vi "Get Disable.vi"(8 "error in (no error)":errorcluster, 11 "S4ACS_GUI in":refnum<class "S4ACS_GUI.lvclass">) -> (0 "error out":errorcluster, 2 "Cluster Disable":T1, 3 "S4ACS_GUI out":refnum<class "S4ACS_GUI.lvclass">)   [LabVIEW 2018, in "S4ACS_GUI.lvclass"]
uses:
  S4ACS_GUI.lvclass
  S4ACS_GUI.lvclass/S4ACS_GUI.ctl
  Acquisition/Acquisition.lvclass
  Instrument/Instrument.lvclass
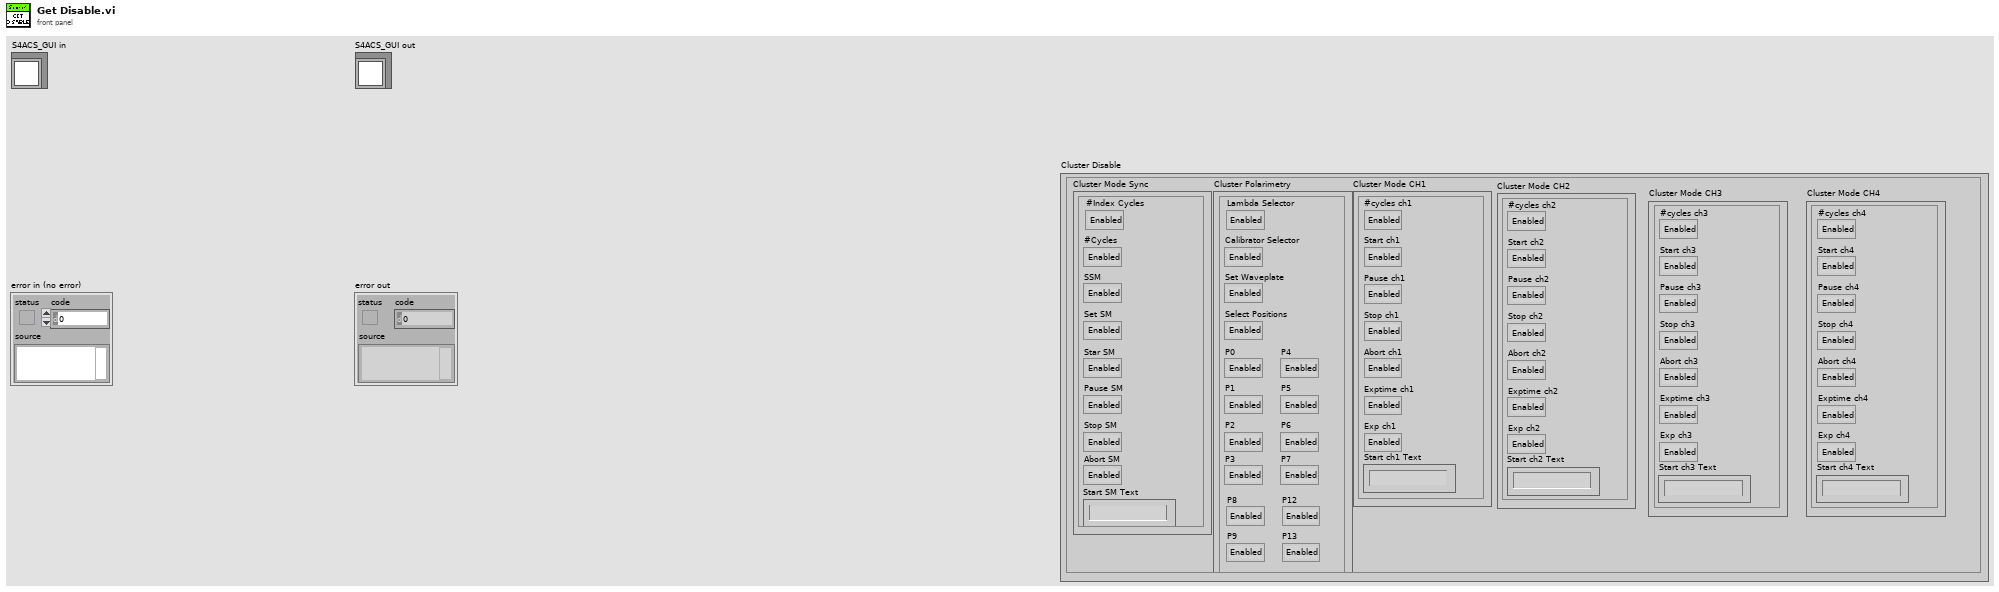
[diagram p1: front panel]
types:
  T1 = cluster{"Cluster Mode Sync":cluster{"#Index Cycles":enum8{"Enabled", "Disabled", "Disabled and Grayed Out"}, "#Cycles":enum8{"Enabled", "Disabled", "Disabled and Grayed Out"}, "SSM":enum8{"Enabled", "Disabled", "Disabled and Grayed Out"}, "Set SM":enum8{"Enabled", "Disabled", "Disabled and Grayed Out"}, "Star SM":enum8{"Enabled", "Disabled", "Disabled and Grayed Out"}, "Pause SM":enum8{"Enabled", "Disabled", "Disabled and Grayed Out"}, "Stop SM":enum8{"Enabled", "Disabled", "Disabled and Grayed Out"}, "Abort SM":enum8{"Enabled", "Disabled", "Disabled and Grayed Out"}, "Start SM Text":string}, "Cluster Polarimetry":cluster{"Lambda Selector":enum8{"Enabled", "Disabled", "Disabled and Grayed Out"}, "Calibrator Selector":enum8{"Enabled", "Disabled", "Disabled and Grayed Out"}, "Set Waveplate":enum8{"Enabled", "Disabled", "Disabled and Grayed Out"}, "Select Positions":enum8{"Enabled", "Disabled", "Disabled and Grayed Out"}, "P0":enum8{"Enabled", "Disabled", "Disabled and Grayed Out"}, "P1":enum8{"Enabled", "Disabled", "Disabled and Grayed Out"}, "P2":enum8{"Enabled", "Disabled", "Disabled and Grayed Out"}, "P3":enum8{"Enabled", "Disabled", "Disabled and Grayed Out"}, "P4":enum8{"Enabled", "Disabled", "Disabled and Grayed Out"}, "P5":enum8{"Enabled", "Disabled", "Disabled and Grayed Out"}, "P6":enum8{"Enabled", "Disabled", "Disabled and Grayed Out"}, "P7":enum8{"Enabled", "Disabled", "Disabled and Grayed Out"}, "P8":enum8{"Enabled", "Disabled", "Disabled and Grayed Out"}, "P9":enum8{"Enabled", "Disabled", "Disabled and Grayed Out"}, "P10":enum8{"Enabled", "Disabled", "Disabled and Grayed Out"}, "P11":enum8{"Enabled", "Disabled", "Disabled and Grayed Out"}, "P12":enum8{"Enabled", "Disabled", "Disabled and Grayed Out"}, "P13":enum8{"Enabled", "Disabled", "Disabled and Grayed Out"}, "P14":enum8{"Enabled", "Disabled", "Disabled and Grayed Out"}, "P15":enum8{"Enabled", "Disabled", "Disabled and Grayed Out"}}, "Cluster Mode CH1":cluster{"#cycles ch1":enum8{"Enabled", "Disabled", "Disabled and Grayed Out"}, "Start ch1":enum8{"Enabled", "Disabled", "Disabled and Grayed Out"}, "Pause ch1":enum8{"Enabled", "Disabled", "Disabled and Grayed Out"}, "Stop ch1":enum8{"Enabled", "Disabled", "Disabled and Grayed Out"}, "Abort ch1":enum8{"Enabled", "Disabled", "Disabled and Grayed Out"}, "Exptime ch1":enum8{"Enabled", "Disabled", "Disabled and Grayed Out"}, "Exp ch1":enum8{"Enabled", "Disabled", "Disabled and Grayed Out"}, "Start ch1 Text":string}, "Cluster Mode CH2":cluster{"#cycles ch2":enum8{"Enabled", "Disabled", "Disabled and Grayed Out"}, "Start ch2":enum8{"Enabled", "Disabled", "Disabled and Grayed Out"}, "Pause ch2":enum8{"Enabled", "Disabled", "Disabled and Grayed Out"}, "Stop ch2":enum8{"Enabled", "Disabled", "Disabled and Grayed Out"}, "Abort ch2":enum8{"Enabled", "Disabled", "Disabled and Grayed Out"}, "Exptime ch2":enum8{"Enabled", "Disabled", "Disabled and Grayed Out"}, "Exp ch2":enum8{"Enabled", "Disabled", "Disabled and Grayed Out"}, "Start ch2 Text":string}, "Cluster Mode CH3":cluster{"#cycles ch3":enum8{"Enabled", "Disabled", "Disabled and Grayed Out"}, "Start ch3":enum8{"Enabled", "Disabled", "Disabled and Grayed Out"}, "Pause ch3":enum8{"Enabled", "Disabled", "Disabled and Grayed Out"}, "Stop ch3":enum8{"Enabled", "Disabled", "Disabled and Grayed Out"}, "Abort ch3":enum8{"Enabled", "Disabled", "Disabled and Grayed Out"}, "Exptime ch3":enum8{"Enabled", "Disabled", "Disabled and Grayed Out"}, "Exp ch3":enum8{"Enabled", "Disabled", "Disabled and Grayed Out"}, "Start ch3 Text":string}, "Cluster Mode CH4":cluster{"#cycles ch4":enum8{"Enabled", "Disabled", "Disabled and Grayed Out"}, "Start ch4":enum8{"Enabled", "Disabled", "Disabled and Grayed Out"}, "Pause ch4":enum8{"Enabled", "Disabled", "Disabled and Grayed Out"}, "Stop ch4":enum8{"Enabled", "Disabled", "Disabled and Grayed Out"}, "Abort ch4":enum8{"Enabled", "Disabled", "Disabled and Grayed Out"}, "Exptime ch4":enum8{"Enabled", "Disabled", "Disabled and Grayed Out"}, "Exp ch4":enum8{"Enabled", "Disabled", "Disabled and Grayed Out"}, "Start ch4 Text":string}}
  T2 = enum8{"Enabled", "Disabled", "Disabled and Grayed Out"}
  T3 = cluster{"#Index Cycles":enum8{"Enabled", "Disabled", "Disabled and Grayed Out"}, "#Cycles":enum8{"Enabled", "Disabled", "Disabled and Grayed Out"}, "SSM":enum8{"Enabled", "Disabled", "Disabled and Grayed Out"}, "Set SM":enum8{"Enabled", "Disabled", "Disabled and Grayed Out"}, "Star SM":enum8{"Enabled", "Disabled", "Disabled and Grayed Out"}, "Pause SM":enum8{"Enabled", "Disabled", "Disabled and Grayed Out"}, "Stop SM":enum8{"Enabled", "Disabled", "Disabled and Grayed Out"}, "Abort SM":enum8{"Enabled", "Disabled", "Disabled and Grayed Out"}, "Start SM Text":string}
  T4 = cluster{"#cycles ch1":enum8{"Enabled", "Disabled", "Disabled and Grayed Out"}, "Start ch1":enum8{"Enabled", "Disabled", "Disabled and Grayed Out"}, "Pause ch1":enum8{"Enabled", "Disabled", "Disabled and Grayed Out"}, "Stop ch1":enum8{"Enabled", "Disabled", "Disabled and Grayed Out"}, "Abort ch1":enum8{"Enabled", "Disabled", "Disabled and Grayed Out"}, "Exptime ch1":enum8{"Enabled", "Disabled", "Disabled and Grayed Out"}, "Exp ch1":enum8{"Enabled", "Disabled", "Disabled and Grayed Out"}, "Start ch1 Text":string}
  T5 = cluster{"#cycles ch2":enum8{"Enabled", "Disabled", "Disabled and Grayed Out"}, "Start ch2":enum8{"Enabled", "Disabled", "Disabled and Grayed Out"}, "Pause ch2":enum8{"Enabled", "Disabled", "Disabled and Grayed Out"}, "Stop ch2":enum8{"Enabled", "Disabled", "Disabled and Grayed Out"}, "Abort ch2":enum8{"Enabled", "Disabled", "Disabled and Grayed Out"}, "Exptime ch2":enum8{"Enabled", "Disabled", "Disabled and Grayed Out"}, "Exp ch2":enum8{"Enabled", "Disabled", "Disabled and Grayed Out"}, "Start ch2 Text":string}
  T6 = cluster{"#cycles ch3":enum8{"Enabled", "Disabled", "Disabled and Grayed Out"}, "Start ch3":enum8{"Enabled", "Disabled", "Disabled and Grayed Out"}, "Pause ch3":enum8{"Enabled", "Disabled", "Disabled and Grayed Out"}, "Stop ch3":enum8{"Enabled", "Disabled", "Disabled and Grayed Out"}, "Abort ch3":enum8{"Enabled", "Disabled", "Disabled and Grayed Out"}, "Exptime ch3":enum8{"Enabled", "Disabled", "Disabled and Grayed Out"}, "Exp ch3":enum8{"Enabled", "Disabled", "Disabled and Grayed Out"}, "Start ch3 Text":string}
  T7 = cluster{"#cycles ch4":enum8{"Enabled", "Disabled", "Disabled and Grayed Out"}, "Start ch4":enum8{"Enabled", "Disabled", "Disabled and Grayed Out"}, "Pause ch4":enum8{"Enabled", "Disabled", "Disabled and Grayed Out"}, "Stop ch4":enum8{"Enabled", "Disabled", "Disabled and Grayed Out"}, "Abort ch4":enum8{"Enabled", "Disabled", "Disabled and Grayed Out"}, "Exptime ch4":enum8{"Enabled", "Disabled", "Disabled and Grayed Out"}, "Exp ch4":enum8{"Enabled", "Disabled", "Disabled and Grayed Out"}, "Start ch4 Text":string}
  T8 = cluster{"Lambda Selector":enum8{"Enabled", "Disabled", "Disabled and Grayed Out"}, "Calibrator Selector":enum8{"Enabled", "Disabled", "Disabled and Grayed Out"}, "Set Waveplate":enum8{"Enabled", "Disabled", "Disabled and Grayed Out"}, "Select Positions":enum8{"Enabled", "Disabled", "Disabled and Grayed Out"}, "P0":enum8{"Enabled", "Disabled", "Disabled and Grayed Out"}, "P1":enum8{"Enabled", "Disabled", "Disabled and Grayed Out"}, "P2":enum8{"Enabled", "Disabled", "Disabled and Grayed Out"}, "P3":enum8{"Enabled", "Disabled", "Disabled and Grayed Out"}, "P4":enum8{"Enabled", "Disabled", "Disabled and Grayed Out"}, "P5":enum8{"Enabled", "Disabled", "Disabled and Grayed Out"}, "P6":enum8{"Enabled", "Disabled", "Disabled and Grayed Out"}, "P7":enum8{"Enabled", "Disabled", "Disabled and Grayed Out"}, "P8":enum8{"Enabled", "Disabled", "Disabled and Grayed Out"}, "P9":enum8{"Enabled", "Disabled", "Disabled and Grayed Out"}, "P10":enum8{"Enabled", "Disabled", "Disabled and Grayed Out"}, "P11":enum8{"Enabled", "Disabled", "Disabled and Grayed Out"}, "P12":enum8{"Enabled", "Disabled", "Disabled and Grayed Out"}, "P13":enum8{"Enabled", "Disabled", "Disabled and Grayed Out"}, "P14":enum8{"Enabled", "Disabled", "Disabled and Grayed Out"}, "P15":enum8{"Enabled", "Disabled", "Disabled and Grayed Out"}}
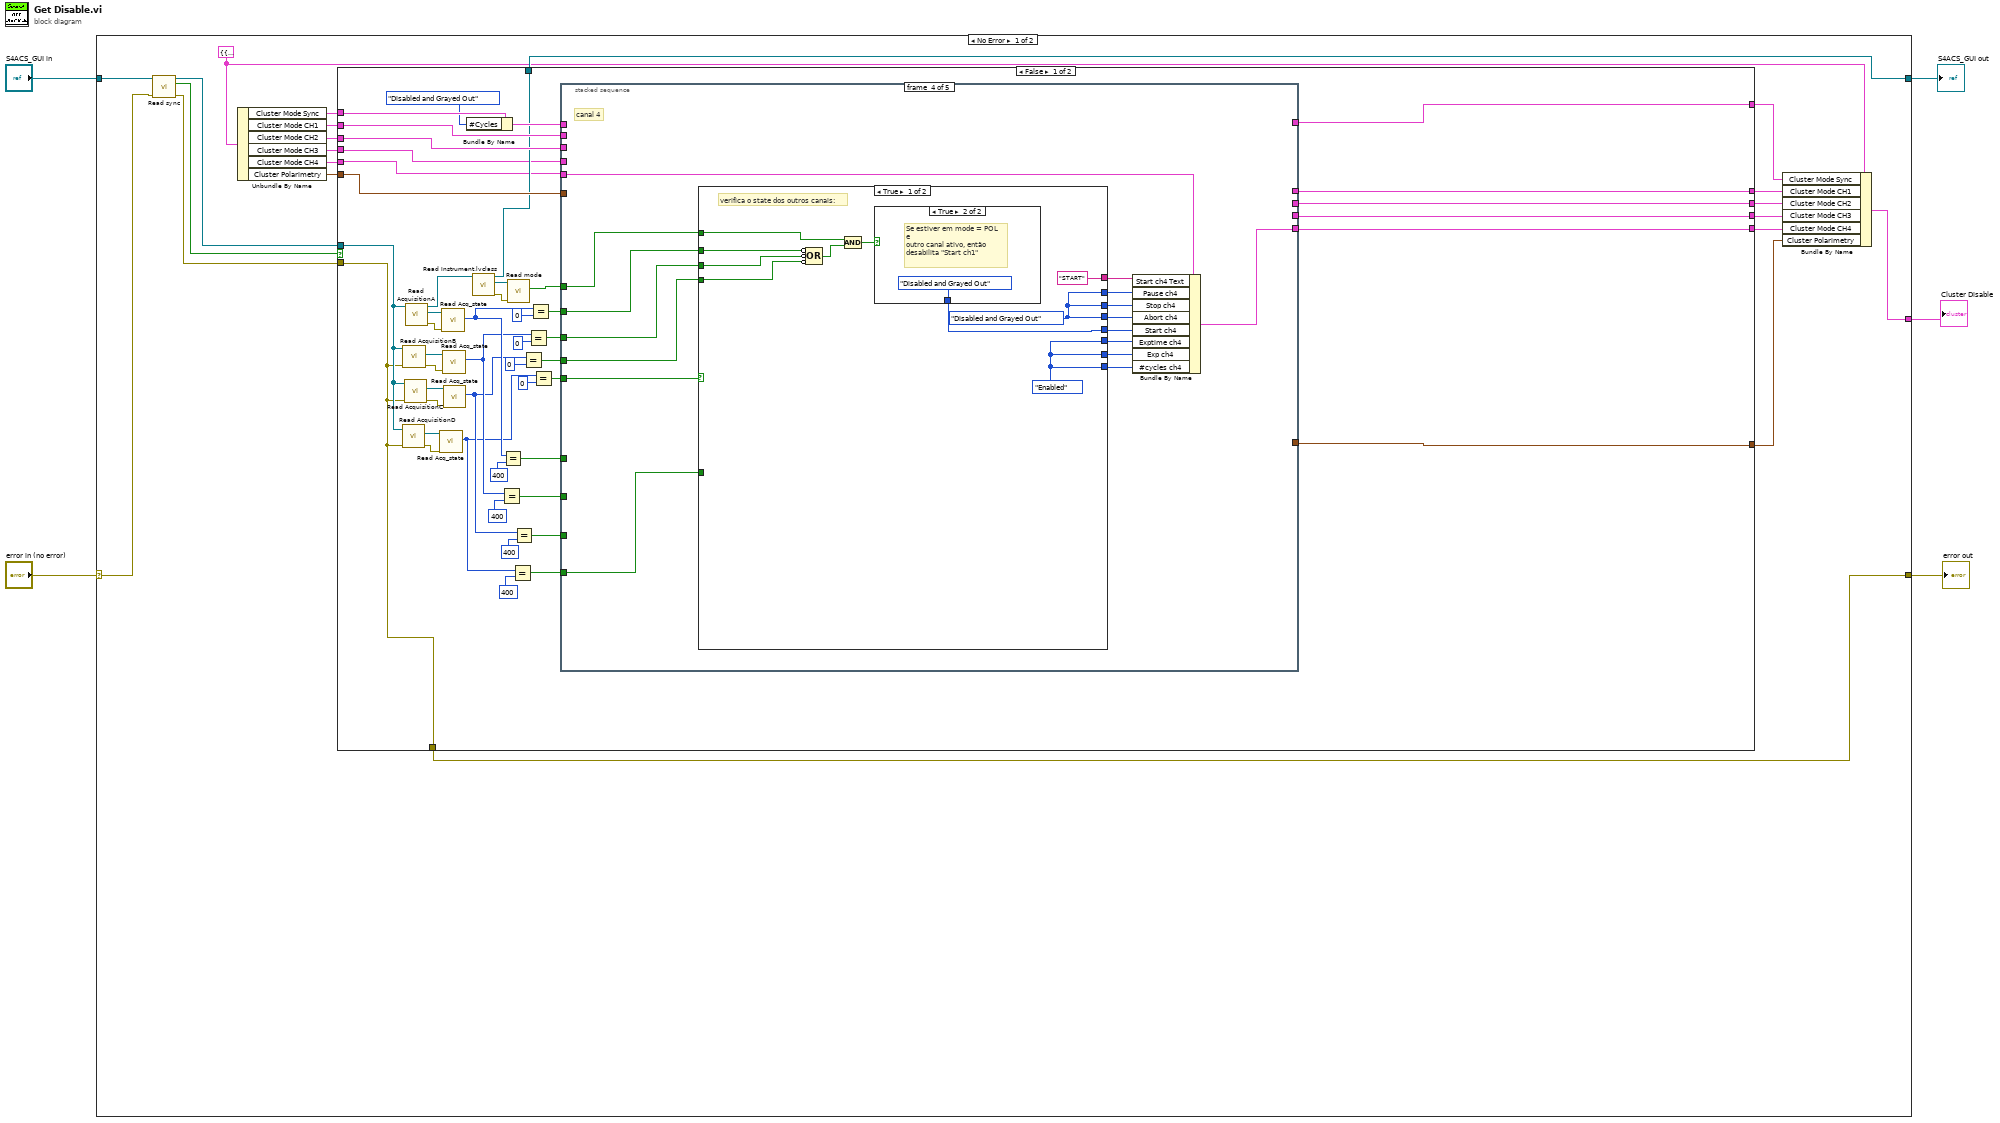
[diagram p0: block diagram]
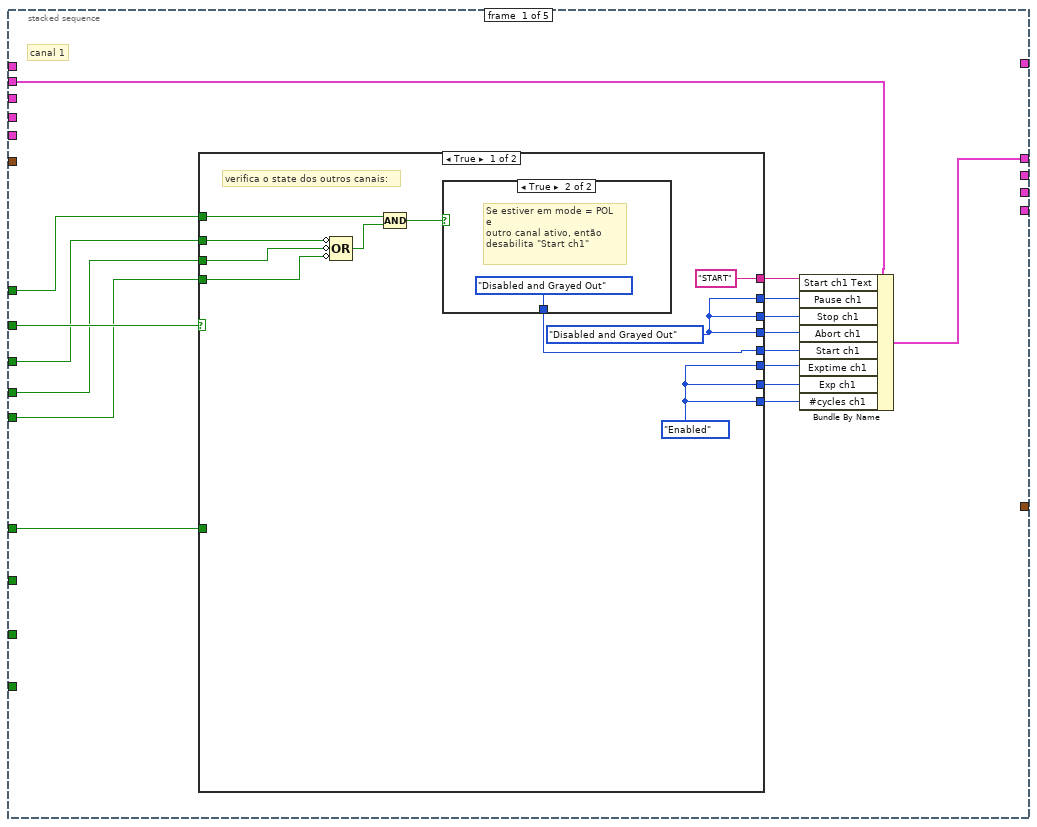
[diagram p2: hidden frame]
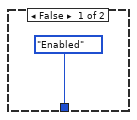
[diagram p3: hidden frame]
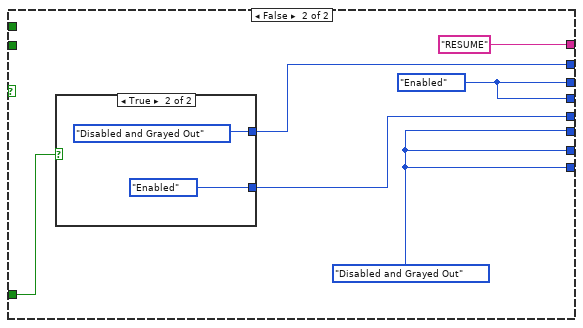
[diagram p4: hidden frame]
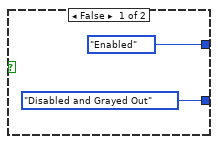
[diagram p5: hidden frame]
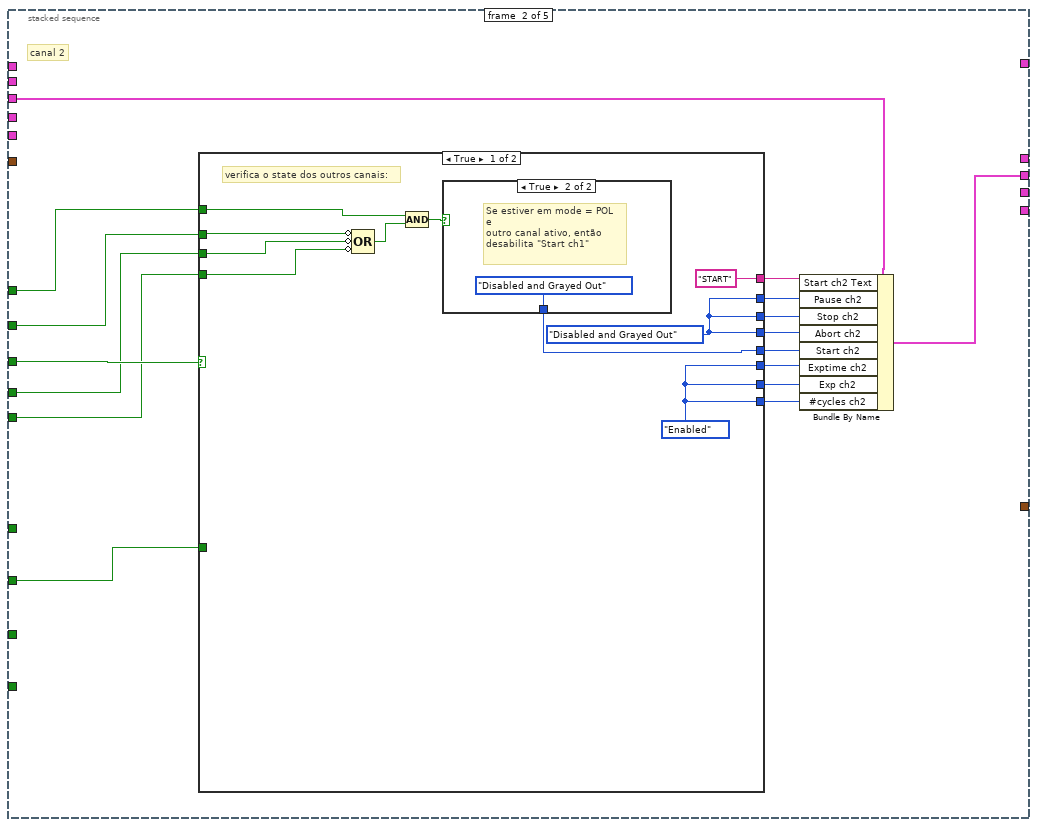
[diagram p6: hidden frame]
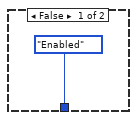
[diagram p7: hidden frame]
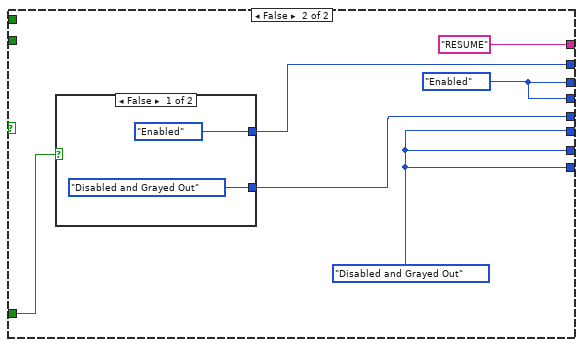
[diagram p8: hidden frame]
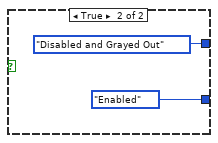
[diagram p9: hidden frame]
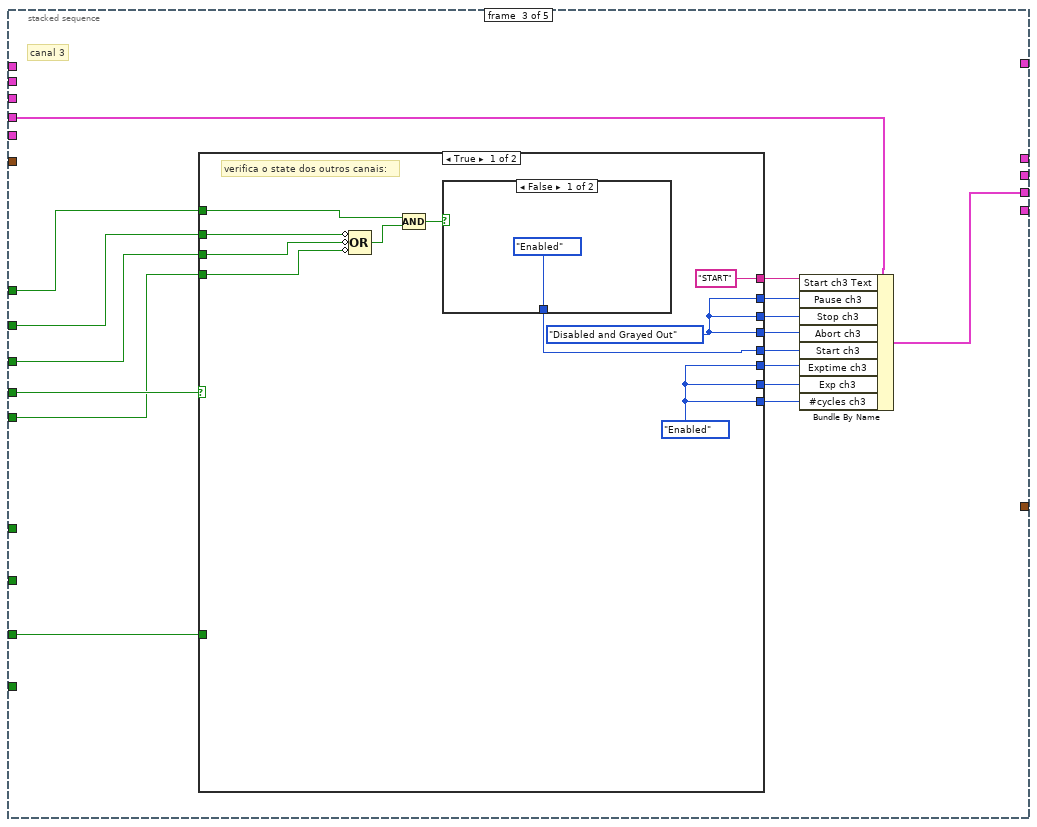
[diagram p10: hidden frame]
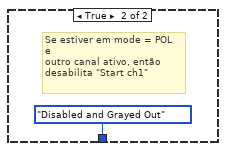
[diagram p11: hidden frame]
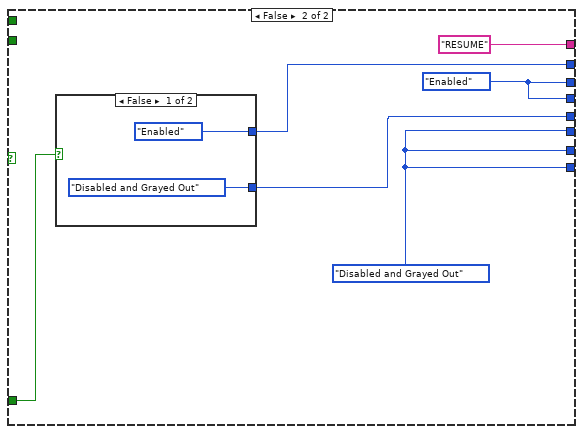
[diagram p12: hidden frame]
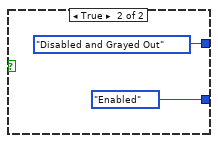
[diagram p13: hidden frame]
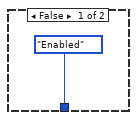
[diagram p14: hidden frame]
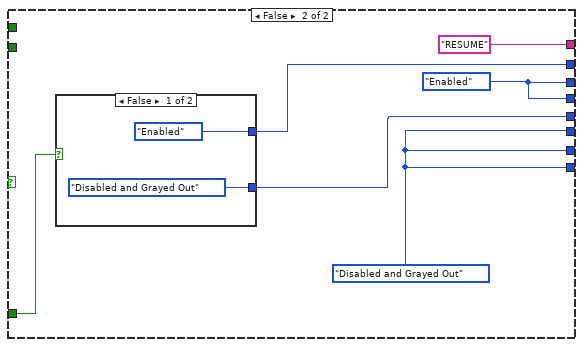
[diagram p15: hidden frame]
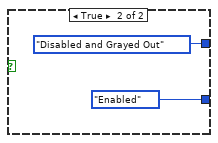
[diagram p16: hidden frame]
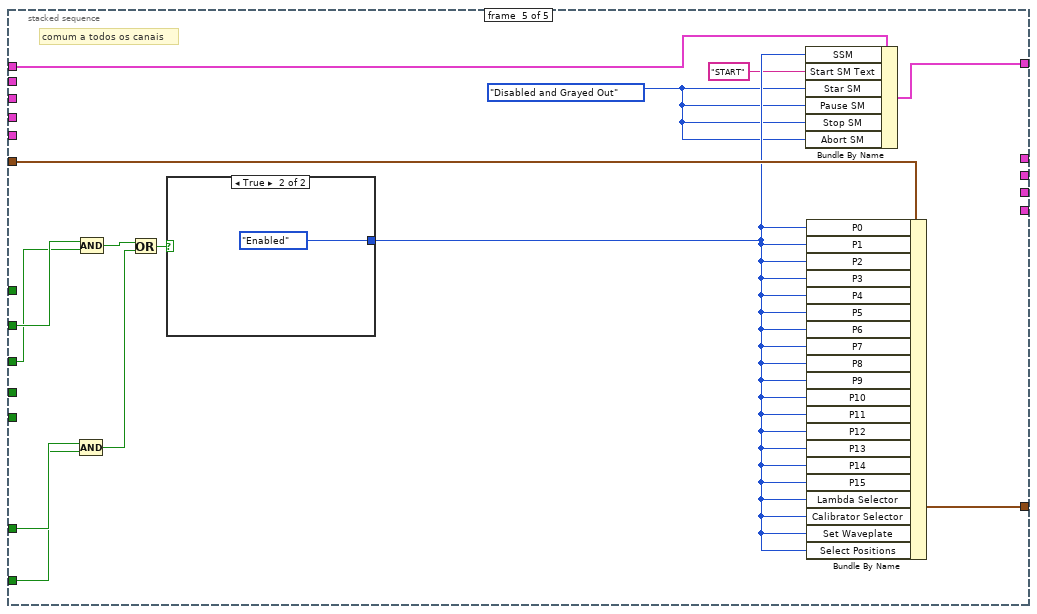
[diagram p17: hidden frame]
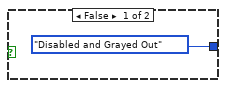
[diagram p18: hidden frame]
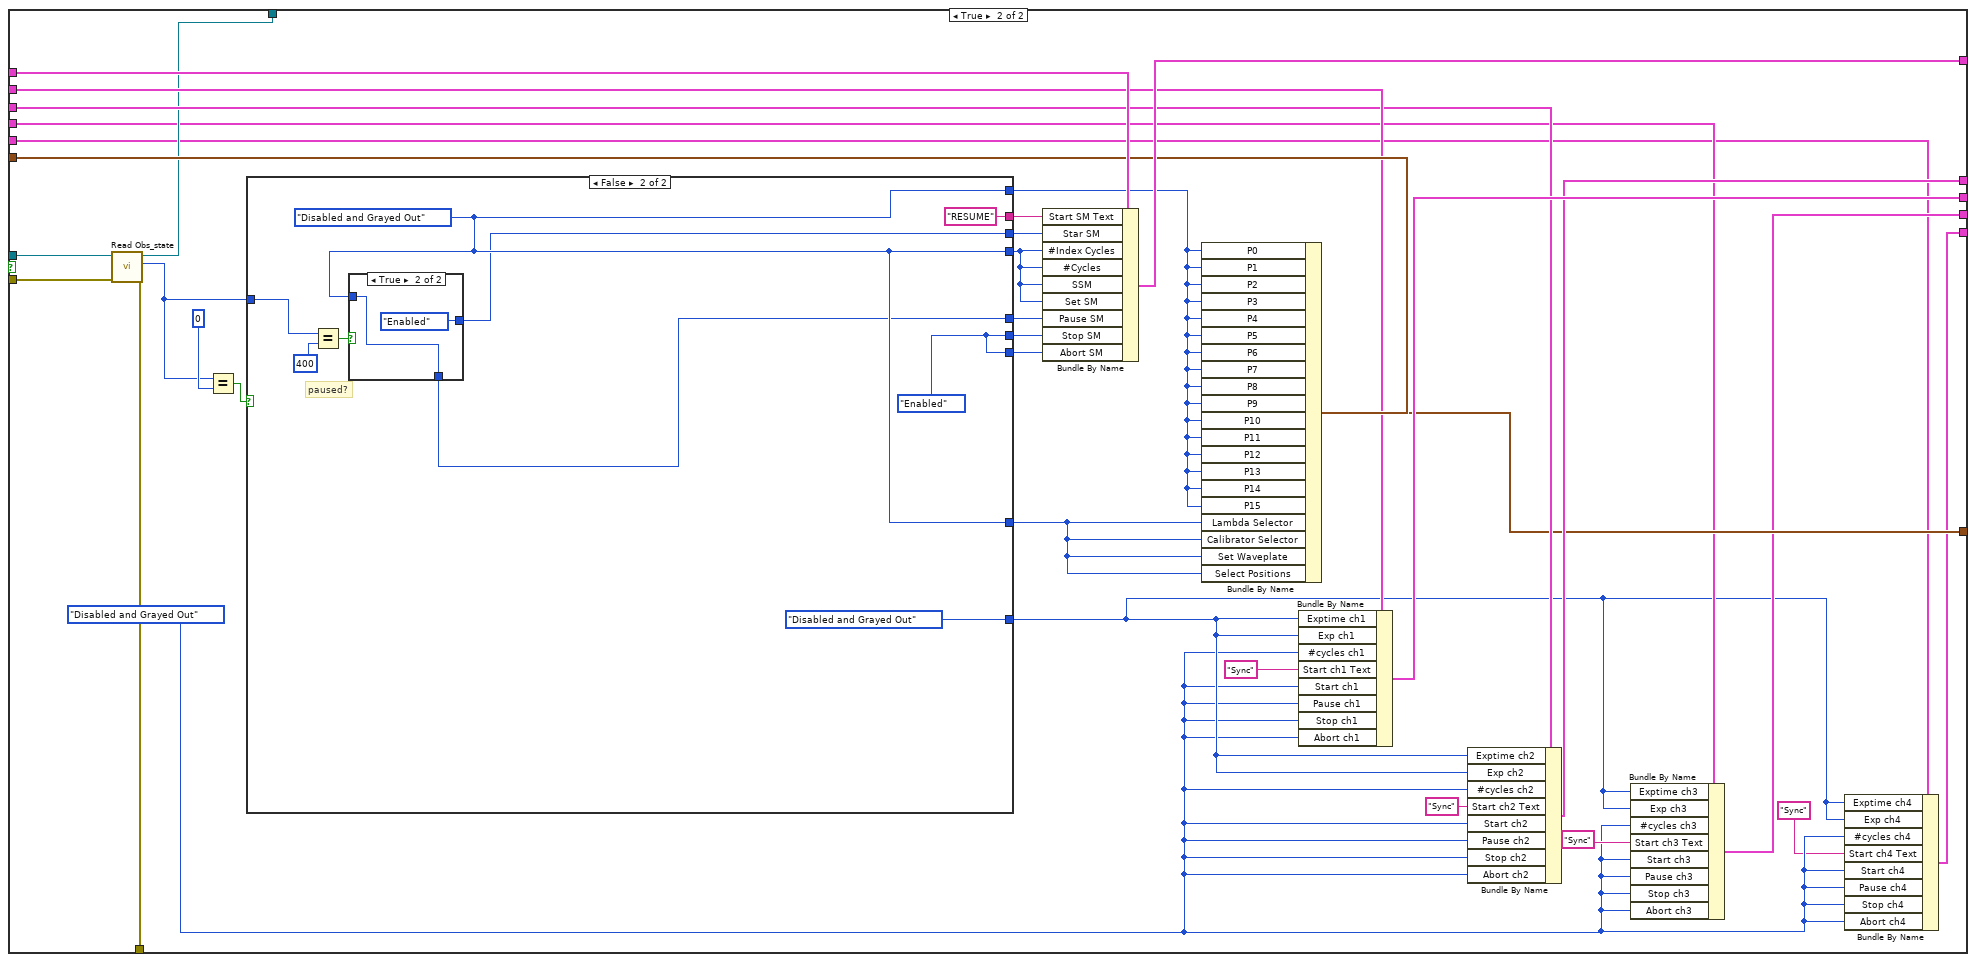
[diagram p19: hidden frame]
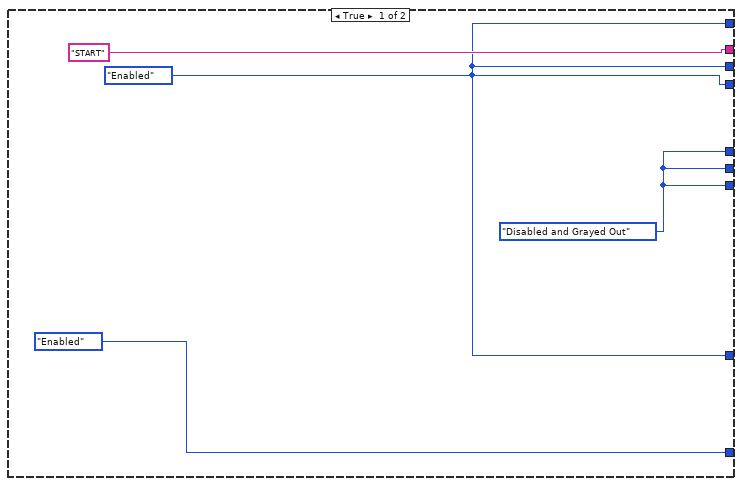
[diagram p20: hidden frame]
diagram:
  n1 = case shown="No Error" "error in (no error)" {
    selector: "error in (no error)" -> [w21 w295]
    tunnel: [w14 w295] -> w4
    tunnel: [w13 w294] -> w2
    tunnel: "S4ACS_GUI in" -> [w22 w294]
    tunnel: [w26 _] -> w1
    frame No Error {
      w12 = T1 {"Cluster Mode Sync"={"#Index Cycles"=enum."Enabled", "#Cycles"=enum."Enabled", "SSM"=enum."Enabled", "Set SM"=enum."Enabled", "Star SM"=enum."Enabled", "Pause SM"=enum."Enabled", "Stop SM"=enum."Enabled", "Abort SM"=enum."Enabled", "Start SM Text"=""}, "Cluster Polarimetry"={"Lambda Selector"=enum."Enabled", "Calibrator Selector"=enum."Enabled", "Set Waveplate"=enum."Enabled", "Select Positions"=enum."Enabled", "P0"=enum."Enabled", "P1"=enum."Enabled", "P2"=enum."Enabled", "P3"=enum."Enabled", "P4"=enum."Enabled", "P5"=enum."Enabled", "P6"=enum."Enabled", "P7"=enum."Enabled", "P8"=enum."Enabled", "P9"=enum."Enabled", "P10"=enum."Enabled", "P11"=enum."Enabled", "P12"=enum."Enabled", "P13"=enum."Enabled", "P14"=enum."Enabled", "P15"=enum."Enabled"}, "Cluster Mode CH1"={"#cycles ch1"=enum."Enabled", "Start ch1"=enum."Enabled", "Pause ch1"=enum."Enabled", "Stop ch1"=enum."Enabled", "Abort ch1"=enum."Enabled", "Exptime ch1"=enum."Enabled", "Exp ch1"=enum."Enabled", "Start ch1 Text"=""}, "Cluster Mode CH2"={"#cycles ch2"=enum."Enabled", "Start ch2"=enum."Enabled", "Pause ch2"=enum."Enabled", "Stop ch2"=enum."Enabled", "Abort ch2"=enum."Enabled", "Exptime ch2"=enum."Enabled", "Exp ch2"=enum."Enabled", "Start ch2 Text"=""}, "Cluster Mode CH3"={"#cycles ch3"=enum."Enabled", "Start ch3"=enum."Enabled", "Pause ch3"=enum."Enabled", "Stop ch3"=enum."Enabled", "Abort ch3"=enum."Enabled", "Exptime ch3"=enum."Enabled", "Exp ch3"=enum."Enabled", "Start ch3 Text"=""}, "Cluster Mode CH4"={"#cycles ch4"=enum."Enabled", "Start ch4"=enum."Enabled", "Pause ch4"=enum."Enabled", "Stop ch4"=enum."Enabled", "Abort ch4"=enum."Enabled", "Exptime ch4"=enum."Enabled", "Exp ch4"=enum."Enabled", "Start ch4 Text"=""}} ("Cluster Disable 2")
      n2 = call-dynamic "Read sync.vi"("error in (no error)"=w21, "S4ACS_GUI in"=w22) -> ("error out"=w25:errorcluster, "sync"=w23:bool, "S4ACS_GUI out"=w24:refnum<class "S4ACS_GUI.lvclass">)  [unwired: 7 in]
      n3 = Unbundle By Name(w12) -> ("Cluster Mode Sync"=w20:T3, "Cluster Mode CH1"=w19:T4, "Cluster Mode CH2"=w18:T5, "Cluster Mode CH3"=w10:T6, "Cluster Mode CH4"=w9:T7, "Cluster Polarimetry"=w11:T8)
      n4 = case shown="False" w23 {
        tunnel: w24 -> [w38 w273]
        tunnel: w25 -> [w37 w272]
        tunnel: w20 -> [w57 w271]
        tunnel: w19 -> [w54 w260]
        tunnel: w18 -> [w52 w257]
        tunnel: [w53 w269] -> w17
        tunnel: [w49 w258] -> w16
        tunnel: w11 -> [w51 w268]
        tunnel: [w50 w256] -> w8
        tunnel: [w48 w259] -> w15
        tunnel: [w37 w255] -> w14
        tunnel: [w47 w254] -> w13
        tunnel: w10 -> [w46 w250]
        tunnel: w9 -> [w45 w245]
        tunnel: [w44 w249] -> w7
        tunnel: [w43 w244] -> w6
        frame False {
          n5 = call-dynamic "Read AcquisitionD.vi"("error in (no error)"=w37, "S4ACS_GUI in"=w38) -> ("error out"=w39:errorcluster, "Acquisition.lvclass"=w40:refnum<class "Acquisition.lvclass">)  [unwired: 7 in, 1 out]
          n6 = call "Read AcquisitionB.vi"("error in (no error)"=w37, "S4ACS_GUI in"=w38) -> ("error out"=w72:errorcluster, "Acquisition.lvclass"=w73:refnum<class "Acquisition.lvclass">)  [unwired: 7 in, 1 out]
          n7 = call-dynamic "Read AcquisitionC.vi"("error in (no error)"=w37, "S4ACS_GUI in"=w38) -> ("error out"=w42:errorcluster, "Acquisition.lvclass"=w41:refnum<class "Acquisition.lvclass">)  [unwired: 7 in, 1 out]
          n8 = call-dynamic "Read AcquisitionA.vi"("S4ACS_GUI in"=w38) -> ("error out"=w74:errorcluster, "Acquisition.lvclass"=w75:refnum<class "Acquisition.lvclass">, "S4ACS_GUI out"=w58:refnum<class "S4ACS_GUI.lvclass">)  [unwired: 8 in]
          n9 = call-dynamic "Read Acq_state.vi"("error in (no error)"=w39, "Acquisition in"=w40) -> ("Acq_state"=w29:u32)  [unwired: 7 in, 2 out]
          n10 = call-dynamic "Read Acq_state.vi"("error in (no error)"=w74, "Acquisition in"=w75) -> ("Acq_state"=w65:u32)  [unwired: 7 in, 2 out]
          n11 = call-dynamic "Read Acq_state.vi"("error in (no error)"=w72, "Acquisition in"=w73) -> ("Acq_state"=w62:u32)  [unwired: 7 in, 2 out]
          n12 = call-dynamic "Read Acq_state.vi"("error in (no error)"=w42, "Acquisition in"=w41) -> ("Acq_state"=w30:u32)  [unwired: 7 in, 2 out]
          n13 = Bundle By Name(cluster=w57, "#Cycles"=T2."Disabled and Grayed Out" ("Disabled")) -> (w55:T3)
          n14 = call "Read Instrument.lvclass.vi"("S4ACS_GUI in"=w58) -> ("error out"=w60:errorcluster, "Instrument.lvclass"=w61:refnum<class "Instrument.lvclass">, "S4ACS_GUI out"=w47:refnum<class "S4ACS_GUI.lvclass">)  [unwired: 8 in]
          n15 = Equal?(x=w62, y=u32 400) -> (x = y?=w66:bool)
          n16 = Equal?(x=w65, y=u32 400) -> (x = y?=w67:bool)
          n17 = call-dynamic "Read mode.vi"("error in (no error)"=w60, "Instrument in"=w61) -> ("mode"=w59:bool)  [unwired: 7 in, 2 out]
          n18 = Equal?(x=w29, y=u32 400) -> (x = y?=w27:bool)
          n19 = Equal?(x=w30, y=u32 400) -> (x = y?=w28:bool)
          n20 = Equal?(x=w30, y=u32 0) -> (x = y?=w34:bool)
          n21 = Equal?(x=w62, y=u32 0) -> (x = y?=w64:bool)
          n22 = Equal?(x=w65, y=u32 0) -> (x = y?=w70:bool)
          n23 = Equal?(x=w29, y=u32 0) -> (x = y?=w35:bool)
          n24 = stacked-sequence {
            tunnel: w70 -> [w91 w118 w158 w196 w241]
            tunnel: w67 -> [w90 _ _ _ w239]
            tunnel: w66 -> [_ w116 _ _ w238]
            tunnel: w64 -> [w88 w117 w155 w192 w240]
            tunnel: w59 -> [w89 w129 w167 w205 _]
            tunnel: w55 -> [_ _ _ _ w232]
            tunnel: w54 -> [w87 _ _ _ _]
            tunnel: [_ _ _ _ w230] -> w53
            tunnel: [w78 _ _ _ _] -> w49
            tunnel: w52 -> [_ w120 _ _ _]
            tunnel: w51 -> [_ _ _ _ w234]
            tunnel: [_ _ _ _ w233] -> w50
            tunnel: [_ w119 _ _ _] -> w48
            tunnel: w46 -> [_ _ w157 _ _]
            tunnel: w45 -> [_ _ _ w195 _]
            tunnel: [_ _ w156 _ _] -> w44
            tunnel: [_ _ _ w194 _] -> w43
            tunnel: w34 -> [w77 w115 w154 w191 _]
            tunnel: w35 -> [w76 w114 w153 w193 _]
            tunnel: w28 -> [_ _ w152 _ _]
            tunnel: w27 -> [_ _ _ w190 _]
            frame #0 {
              # "canal 1"
              n25 = case shown="True" w91 {
                tunnel: w90 -> [_ w109]
                tunnel: w89 -> [w100 _]
                tunnel: w88 -> [w95 _]
                tunnel: ["START" ("Caption.Text") "RESUME" ("Caption.Text")] -> w86
                tunnel: [w98 w106] -> w85
                tunnel: [w98 w104] -> w84
                tunnel: [w98 w104] -> w83
                tunnel: [w97 w107] -> w82
                tunnel: [w96 w105] -> w81
                tunnel: [w96 w105] -> w80
                tunnel: [w96 w105] -> w79
                tunnel: w77 -> [w94 _]
                tunnel: w76 -> [w93 _]
                frame True {
                  w98 = T2."Disabled and Grayed Out" ("Disabled")
                  w96 = T2."Enabled" ("Disabled")
                  # "verifica o state dos outros canais:"
                  n26 = Compound Arithmetic op=OR(invert w95, invert w94, invert w93) -> (w92:bool)
                  n27 = Compound Arithmetic op=AND(w100, w92) -> (w101:bool)
                  n28 = case shown="True" w101 {
                    tunnel: [T2."Enabled" ("Disabled") T2."Disabled and Grayed Out" ("Disabled")] -> w97
                    frame False {
                    }
                    frame True {
                      # "Se estiver em mode = POL\ne\noutro canal ativo, então\ndesabilita \"Start ch1\""
                    }
                  }
                }
                frame False {
                  w104 = T2."Enabled" ("Disabled")
                  w105 = T2."Disabled and Grayed Out" ("Disabled")
                  n29 = case shown="True" w109 {
                    tunnel: [T2."Enabled" ("Disabled") T2."Disabled and Grayed Out" ("Disabled")] -> w106
                    tunnel: [T2."Disabled and Grayed Out" ("Disabled") T2."Enabled" ("Disabled")] -> w107
                    frame False {
                    }
                    frame True {
                    }
                  }
                }
              }
              n30 = Bundle By Name(cluster=w87, "Start ch1 Text"=w86, "Pause ch1"=w85, "Stop ch1"=w84, "Abort ch1"=w83, "Start ch1"=w82, "Exptime ch1"=w81, "Exp ch1"=w80, "#cycles ch1"=w79) -> (w78:T4)
            }
            frame #1 {
              # "canal 2"
              n31 = case shown="True" w117 {
                tunnel: w116 -> [_ w147]
                tunnel: w129 -> [w134 _]
                tunnel: w118 -> [w133 _]
                tunnel: ["START" ("Caption.Text") "RESUME" ("Caption.Text")] -> w128
                tunnel: [w138 w145] -> w127
                tunnel: [w138 w142] -> w126
                tunnel: [w138 w142] -> w125
                tunnel: [w137 w143] -> w124
                tunnel: [w136 w144] -> w123
                tunnel: [w136 w144] -> w122
                tunnel: [w136 w144] -> w121
                tunnel: w115 -> [w132 _]
                tunnel: w114 -> [w131 _]
                frame True {
                  w138 = T2."Disabled and Grayed Out" ("Disabled")
                  w136 = T2."Enabled" ("Disabled")
                  # "verifica o state dos outros canais:"
                  n32 = Compound Arithmetic op=OR(invert w133, invert w132, invert w131) -> (w135:bool)
                  n33 = Compound Arithmetic op=AND(w134, w135) -> (w130:bool)
                  n34 = case shown="True" w130 {
                    tunnel: [T2."Enabled" ("Disabled") T2."Disabled and Grayed Out" ("Disabled")] -> w137
                    frame False {
                    }
                    frame True {
                      # "Se estiver em mode = POL\ne\noutro canal ativo, então\ndesabilita \"Start ch1\""
                    }
                  }
                }
                frame False {
                  w142 = T2."Enabled" ("Disabled")
                  w144 = T2."Disabled and Grayed Out" ("Disabled")
                  n35 = case shown="False" w147 {
                    tunnel: [T2."Enabled" ("Disabled") T2."Disabled and Grayed Out" ("Disabled")] -> w145
                    tunnel: [T2."Disabled and Grayed Out" ("Disabled") T2."Enabled" ("Disabled")] -> w143
                    frame False {
                    }
                    frame True {
                    }
                  }
                }
              }
              n36 = Bundle By Name(cluster=w120, "Start ch2 Text"=w128, "Pause ch2"=w127, "Stop ch2"=w126, "Abort ch2"=w125, "Start ch2"=w124, "Exptime ch2"=w123, "Exp ch2"=w122, "#cycles ch2"=w121) -> (w119:T5)
            }
            frame #2 {
              # "canal 3"
              n37 = case shown="True" w154 {
                tunnel: w152 -> [_ w185]
                tunnel: w167 -> [w172 _]
                tunnel: w158 -> [w171 _]
                tunnel: ["START" ("Caption.Text") "RESUME" ("Caption.Text")] -> w166
                tunnel: [w176 w183] -> w165
                tunnel: [w176 w180] -> w164
                tunnel: [w176 w180] -> w163
                tunnel: [w175 w181] -> w162
                tunnel: [w174 w182] -> w161
                tunnel: [w174 w182] -> w160
                tunnel: [w174 w182] -> w159
                tunnel: w155 -> [w170 _]
                tunnel: w153 -> [w169 _]
                frame True {
                  w176 = T2."Disabled and Grayed Out" ("Disabled")
                  w174 = T2."Enabled" ("Disabled")
                  # "verifica o state dos outros canais:"
                  n38 = Compound Arithmetic op=OR(invert w171, invert w170, invert w169) -> (w173:bool)
                  n39 = Compound Arithmetic op=AND(w172, w173) -> (w168:bool)
                  n40 = case shown="False" w168 {
                    tunnel: [T2."Enabled" ("Disabled") T2."Disabled and Grayed Out" ("Disabled")] -> w175
                    frame False {
                    }
                    frame True {
                      # "Se estiver em mode = POL\ne\noutro canal ativo, então\ndesabilita \"Start ch1\""
                    }
                  }
                }
                frame False {
                  w180 = T2."Enabled" ("Disabled")
                  w182 = T2."Disabled and Grayed Out" ("Disabled")
                  n41 = case shown="False" w185 {
                    tunnel: [T2."Enabled" ("Disabled") T2."Disabled and Grayed Out" ("Disabled")] -> w183
                    tunnel: [T2."Disabled and Grayed Out" ("Disabled") T2."Enabled" ("Disabled")] -> w181
                    frame False {
                    }
                    frame True {
                    }
                  }
                }
              }
              n42 = Bundle By Name(cluster=w157, "Start ch3 Text"=w166, "Pause ch3"=w165, "Stop ch3"=w164, "Abort ch3"=w163, "Start ch3"=w162, "Exptime ch3"=w161, "Exp ch3"=w160, "#cycles ch3"=w159) -> (w156:T6)
            }
            frame #3 {
              # "canal 4"
              n43 = case shown="True" w193 {
                tunnel: w190 -> [_ w223]
                tunnel: w205 -> [w210 _]
                tunnel: w196 -> [w209 _]
                tunnel: ["START" ("Caption.Text") "RESUME" ("Caption.Text")] -> w204
                tunnel: [w214 w221] -> w203
                tunnel: [w214 w218] -> w202
                tunnel: [w214 w218] -> w201
                tunnel: [w213 w219] -> w200
                tunnel: [w212 w220] -> w199
                tunnel: [w212 w220] -> w198
                tunnel: [w212 w220] -> w197
                tunnel: w192 -> [w208 _]
                tunnel: w191 -> [w207 _]
                frame True {
                  w214 = T2."Disabled and Grayed Out" ("Disabled")
                  w212 = T2."Enabled" ("Disabled")
                  # "verifica o state dos outros canais:"
                  n44 = Compound Arithmetic op=OR(invert w209, invert w208, invert w207) -> (w211:bool)
                  n45 = Compound Arithmetic op=AND(w210, w211) -> (w206:bool)
                  n46 = case shown="True" w206 {
                    tunnel: [T2."Enabled" ("Disabled") T2."Disabled and Grayed Out" ("Disabled")] -> w213
                    frame False {
                    }
                    frame True {
                      # "Se estiver em mode = POL\ne\noutro canal ativo, então\ndesabilita \"Start ch1\""
                    }
                  }
                }
                frame False {
                  w218 = T2."Enabled" ("Disabled")
                  w220 = T2."Disabled and Grayed Out" ("Disabled")
                  n47 = case shown="False" w223 {
                    tunnel: [T2."Enabled" ("Disabled") T2."Disabled and Grayed Out" ("Disabled")] -> w221
                    tunnel: [T2."Disabled and Grayed Out" ("Disabled") T2."Enabled" ("Disabled")] -> w219
                    frame False {
                    }
                    frame True {
                    }
                  }
                }
              }
              n48 = Bundle By Name(cluster=w195, "Start ch4 Text"=w204, "Pause ch4"=w203, "Stop ch4"=w202, "Abort ch4"=w201, "Start ch4"=w200, "Exptime ch4"=w199, "Exp ch4"=w198, "#cycles ch4"=w197) -> (w194:T7)
            }
            frame #4 {
              w228 = T2."Disabled and Grayed Out" ("Disabled")
              # "comum a todos os canais"
              n49 = Compound Arithmetic op=AND(w239, w238) -> (w235:bool)
              n50 = Compound Arithmetic op=AND(w241, w240) -> (w236:bool)
              n51 = Or(x=w236, y=w235) -> (x .or. y?=w237:bool)
              n52 = case shown="True" w237 {
                tunnel: [T2."Disabled and Grayed Out" ("Disabled") T2."Enabled" ("Disabled")] -> w231
                frame False {
                }
                frame True {
                }
              }
              n53 = Bundle By Name(cluster=w232, "SSM"=w231, "Start SM Text"="START", "Star SM"=w228, "Pause SM"=w228, "Stop SM"=w228, "Abort SM"=w228) -> (w230:T3)
              n54 = Bundle By Name(cluster=w234, "P0"=w231, "P1"=w231, "P2"=w231, "P3"=w231, "P4"=w231, "P5"=w231, "P6"=w231, "P7"=w231, "P8"=w231, "P9"=w231, "P10"=w231, "P11"=w231, "P12"=w231, "P13"=w231, "P14"=w231, "P15"=w231, "Lambda Selector"=w231, "Calibrator Selector"=w231, "Set Waveplate"=w231, "Select Positions"=w231) -> (w233:T8)
            }
          }
        }
        frame True {
          w247 = T2."Disabled and Grayed Out" ("Disabled")
          n55 = call-dynamic "Read Obs_state.vi"("error in (no error)"=w272, "S4ACS_GUI in"=w273) -> ("error out"=w255:errorcluster, "Obs_state"=w274:u32, "S4ACS_GUI out"=w254:refnum<class "S4ACS_GUI.lvclass">)  [unwired: 7 in]
          n56 = Equal?(x=w274, y=u32 0) -> (x = y?=w275:bool)
          n57 = case shown="False" w275 {
            tunnel: w274 -> [_ w288]
            tunnel: ["START" ("Caption.Text") "RESUME" ("Caption.Text")] -> w270
            tunnel: [w279 w285] -> w267
            tunnel: [w279 w285] -> w266
            tunnel: [w279 w285] -> w265
            tunnel: [w278 w284] -> w264
            tunnel: [w278 w284] -> w263
            tunnel: [w278 w283] -> w262
            tunnel: [w279 w282] -> w261
            tunnel: [T2."Enabled" ("Disabled") T2."Disabled and Grayed Out" ("Disabled")] -> w248
            frame True {
              w278 = T2."Disabled and Grayed Out" ("Disabled")
              w279 = T2."Enabled" ("Disabled")
            }
            frame False {
              w284 = T2."Enabled" ("Disabled")
              w285 = T2."Disabled and Grayed Out" ("Disabled")
              # "paused?"
              n58 = Equal?(x=w288, y=u32 400) -> (x = y?=w289:bool)
              n59 = case shown="True" w289 {
                tunnel: w285 -> [w291 w292]
                tunnel: [w291 T2."Enabled" ("Disabled")] -> w282
                tunnel: [T2."Enabled" ("Disabled") w292] -> w283
                frame False {
                }
                frame True {
                }
              }
            }
          }
          n60 = Bundle By Name(cluster=w271, "Start SM Text"=w270, "Star SM"=w261, "#Index Cycles"=w266, "#Cycles"=w266, "SSM"=w266, "Set SM"=w266, "Pause SM"=w262, "Stop SM"=w264, "Abort SM"=w263) -> (w269:T3)
          n61 = Bundle By Name(cluster=w268, "P0"=w267, "P1"=w267, "P2"=w267, "P3"=w267, "P4"=w267, "P5"=w267, "P6"=w267, "P7"=w267, "P8"=w267, "P9"=w267, "P10"=w267, "P11"=w267, "P12"=w267, "P13"=w267, "P14"=w267, "P15"=w267, "Lambda Selector"=w265, "Calibrator Selector"=w265, "Set Waveplate"=w265, "Select Positions"=w265) -> (w256:T8)
          n62 = Bundle By Name(cluster=w260, "Exptime ch1"=w248, "Exp ch1"=w248, "#cycles ch1"=w247, "Start ch1 Text"="Sync", "Start ch1"=w247, "Pause ch1"=w247, "Stop ch1"=w247, "Abort ch1"=w247) -> (w259:T4)
          n63 = Bundle By Name(cluster=w257, "Exptime ch2"=w248, "Exp ch2"=w248, "#cycles ch2"=w247, "Start ch2 Text"="Sync", "Start ch2"=w247, "Pause ch2"=w247, "Stop ch2"=w247, "Abort ch2"=w247) -> (w258:T5)
          n64 = Bundle By Name(cluster=w250, "Exptime ch3"=w248, "Exp ch3"=w248, "#cycles ch3"=w247, "Start ch3 Text"="Sync" ("Start ch2 Text"), "Start ch3"=w247, "Pause ch3"=w247, "Stop ch3"=w247, "Abort ch3"=w247) -> (w249:T6)
          n65 = Bundle By Name(cluster=w245, "Exptime ch4"=w248, "Exp ch4"=w248, "#cycles ch4"=w247, "Start ch4 Text"="Sync" ("Start ch2 Text"), "Start ch4"=w247, "Pause ch4"=w247, "Stop ch4"=w247, "Abort ch4"=w247) -> (w244:T7)
        }
      }
      n66 = Bundle By Name(cluster=w12, "Cluster Mode Sync"=w17, "Cluster Mode CH1"=w16, "Cluster Mode CH2"=w15, "Cluster Mode CH3"=w7, "Cluster Mode CH4"=w6, "Cluster Polarimetry"=w8) -> (w26:T1)
    }
    frame Error {
    }
  }
  "error out" <- w4
  "S4ACS_GUI out" <- w2
  "Cluster Disable" <- w1
